vi "Test Coffee Shop Removed Barista not Listed.vi"(8 "error in (no error)":errorcluster, 11 "Coffee Shop Test In":refnum<class "Coffee Shop Test.lvclass">=refnum) -> (0 "error out":errorcluster, 3 "Coffee Shop Test Out":refnum<class "Coffee Shop Test.lvclass">)   [LabVIEW 2020, in "Coffee Shop Test.lvclass"]
uses:
  Coffee Shop Test.lvclass
  Processes/Coffee Shop/Coffee Shop.lvclass
  <vilib>/Astemes/Triarc Framework/Process/Process.lvclass
  C:/Program Files (x86)/National Instruments/LabVIEW 2020/vi.lib/Astemes/Triarc Framework/Application/Application.lvclass
  C:/Program Files (x86)/National Instruments/LabVIEW 2020/vi.lib/Astemes/Triarc Framework/Process/Process.lvclass
  C:/Program Files (x86)/National Instruments/LabVIEW 2020/vi.lib/Astemes/Triarc Framework/Base/Base.lvclass
  C:/Program Files (x86)/National Instruments/LabVIEW 2020/vi.lib/Astemes/Triarc Framework/Error Handler Interface/Error Handler Interface.lvclass
  C:/Program Files (x86)/National Instruments/LabVIEW 2020/vi.lib/Astemes/Triarc Framework/Logging/Logging.lvclass
  C:/Program Files (x86)/National Instruments/LabVIEW 2020/vi.lib/Astemes/Triarc Framework/Async Handler/Async Handler.lvclass
  C:/git/astemes-triarc-examples/source/Coffee Shop/Processes/Coffee Shop/Coffee Shop.lvclass
  a7accd14-09a5-49bc-9eb5-7bfb84623754.vi
  <vilib>/Astemes/LUnit/Test Case.lvclass
  C:/Program Files (x86)/National Instruments/LabVIEW 2020/vi.lib/Astemes/LUnit/Test Case.lvclass
  C:/Program Files (x86)/National Instruments/LabVIEW 2020/vi.lib/Astemes/LUnit/LUnit Runnable.lvclass
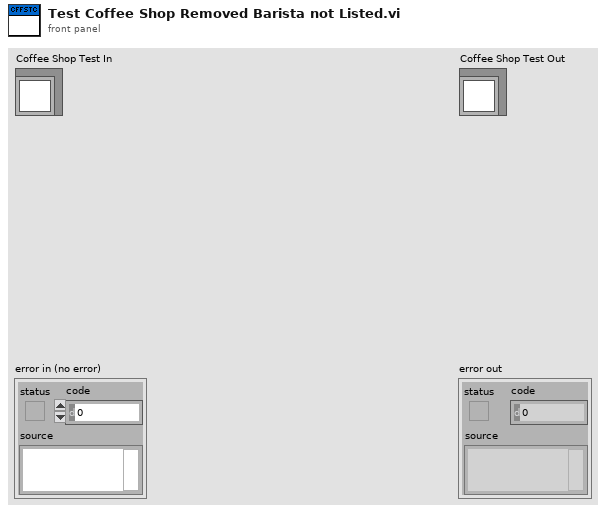
[diagram p1: front panel]
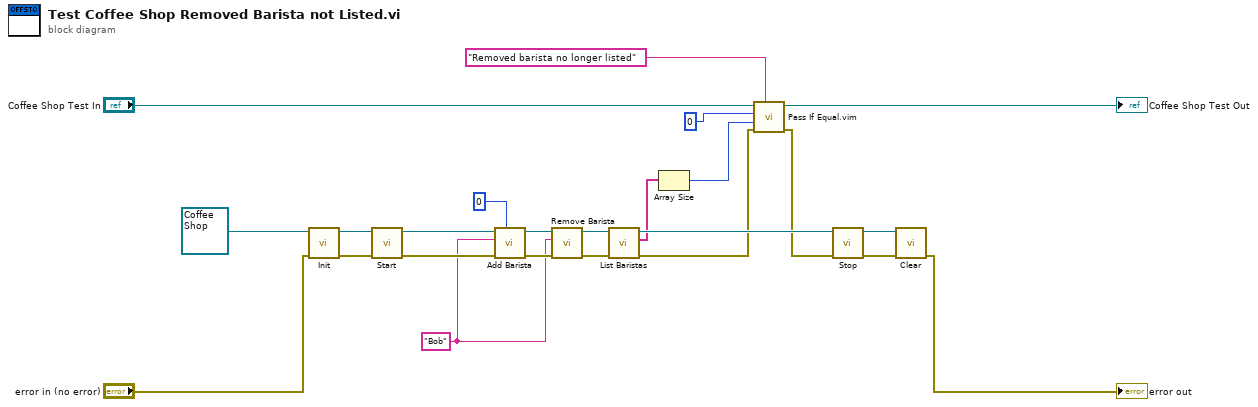
[diagram p0: block diagram]
diagram:
  w8 = "Bob" ("Name")
  n1 = call-dynamic "Init.vi"("error in (no error)"="error in (no error)", "Process In"=refnum<class "Coffee Shop.lvclass"> refnum ("Coffee Shop.lvclass")) -> ("error out"=w22:errorcluster, "Process Out"=w23:refnum<class "Coffee Shop.lvclass">)  [unwired: 8 in]
  n2 = call <vilib>:"Start.vi"("error in (no error)"=w22, "Process In"=w23) -> ("error out"=w17:errorcluster, "Process Out"=w16:refnum<class "Coffee Shop.lvclass">)  [unwired: 7 in, 1 out]
  n3 = call "Add Barista.vi"("Time Scale [ms]"=u32 0, "error in (no error)"=w17, "Name"=w8, "Coffee Shop in"=w16) -> ("error out"=w18:errorcluster, "Coffee Shop out"=w10:refnum<class "Coffee Shop.lvclass">)  [unwired: 6 in]
  n4 = call "Remove Barista.vi"("error in (no error)"=w18, "Name"=w8, "Coffee Shop In"=w10) -> ("error out"=w11:errorcluster, "Coffee Shop Out"=w9:refnum<class "Coffee Shop.lvclass">)  [unwired: 7 in]
  n5 = call "List Baristas.vi"("error in (no error)"=w11, "Coffee Shop in"=w9) -> ("error out"=w5:errorcluster, "Names"=w4:string[], "Coffee Shop out"=w12:refnum<class "Coffee Shop.lvclass">)  [unwired: 7 in]
  n6 = Array Size(array=w4) -> (size(s)=w2:i32)
  n7 = call "Pass If Equal.vim"("Description"="Removed barista no longer listed", "error in (no error)"=w5, "Actual"=w2, "Expected"=0 ("size(s)"), "LUnit Test Case In"="Coffee Shop Test In") -> ("error out"=w7:errorcluster, "LUnit Test Case Out"=→"Coffee Shop Test Out":refnum<class "Test Case.lvclass">)  [unwired: 5 in]
  n8 = call <vilib>:"Stop.vi"("error in (no error)"=w7, "Process In"=w12) -> ("error out"=w20:errorcluster, "Process Out"=w21:refnum<class "Coffee Shop.lvclass">)  [unwired: 7 in, 1 out]
  n9 = call-dynamic "Clear.vi"("error in (no error)"=w20, "Application In"=w21) -> ("error out"=→"error out":errorcluster)  [unwired: 9 in]
